vi "Find MAX Run.vi"(8 "error in (no error)":errorcluster, 10 "RUNSELECT (Most Recent, First, ALL)":string, 11 "Field Information":T1[](array[typedef])) -> (0 "error out":errorcluster, 3 "Field Information 2":T1[](array[typedef]))   [LabVIEW 2011]
uses:
  www/cgi-bin/_cgi-lib/TDM_INDEX Record.ctl
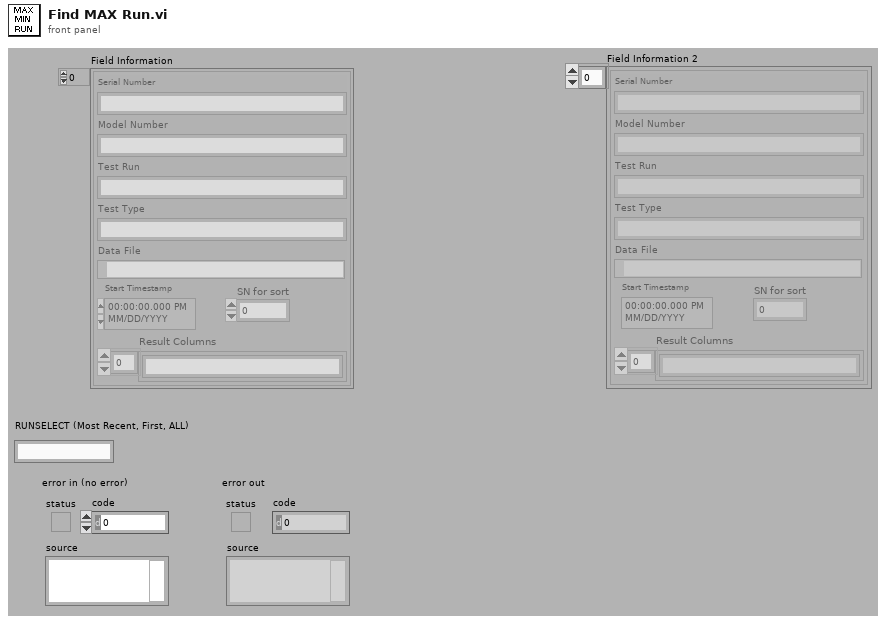
[diagram p1: front panel]
types:
  T1 = typedef "TDM_INDEX Record.ctl" = cluster{"Model Number":string, "SN for sort":i32, "Test Type":string, "Test Run":string, "Serial Number":string, "Start Timestamp":timestamp, "Data File":path, "Result Columns":string[]}
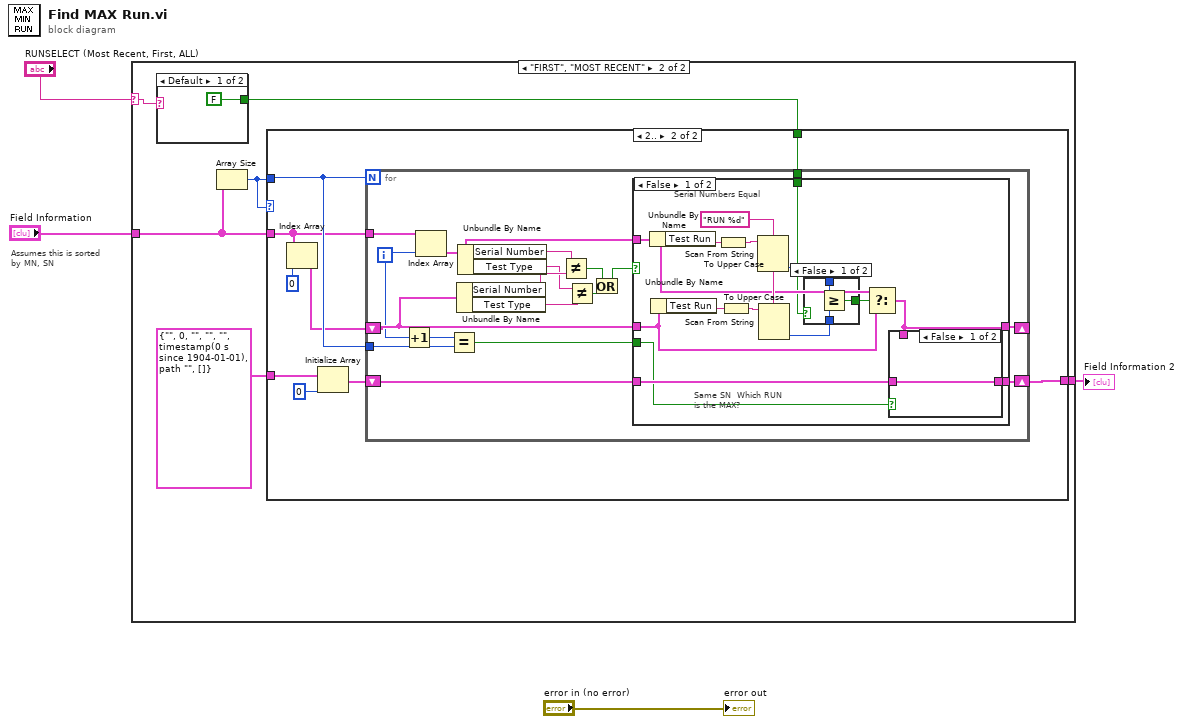
[diagram p0: block diagram]
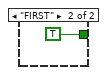
[diagram p3: hidden frame]
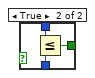
[diagram p5: hidden frame]
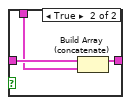
[diagram p6: hidden frame]
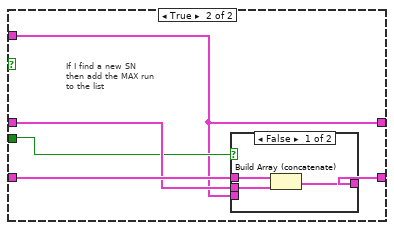
[diagram p7: hidden frame]
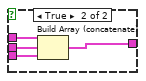
[diagram p8: hidden frame]
diagram:
  # "Assumes this is sorted \nby MN, SN"
  n1 = case shown="\"FIRST\", \"MOST RECENT\"" "RUNSELECT (Most Recent, First, ALL)" {
    selector: "RUNSELECT (Most Recent, First, ALL)" -> [_ w7]
    tunnel: [w5 w10] -> w3
    tunnel: "Field Information" -> [w5 w9]
    frame "ALL", Default {
    }
    frame "FIRST", "MOST RECENT" {
      n2 = case shown="Default" w7 {
        tunnel: [FALSE TRUE] -> w6
        frame Default {
        }
        frame "FIRST" {
        }
      }
      n3 = Array Size(array=w9) -> (size(s)=w8:i32)
      n4 = case shown="2.." w8 {
        tunnel: T1 {"Model Number"="", "SN for sort"=0, "Test Type"="", "Test Run"="", "Serial Number"="", "Start Timestamp"=timestamp(0 s since 1904-01-01), "Data File"=path "", "Result Columns"=[]} ("TDM_INDEX Record") -> [_ w23]
        tunnel: [w14 w20] -> w10
        tunnel: w9 -> [w14 w18]
        tunnel: w8 -> [_ w19]
        tunnel: w6 -> [_ w15]
        frame Default {
          # "If there are 0 or 1 elements no sorting is needed."
        }
        frame 2.. {
          n5 = Index Array(array=w18, index=0) -> (element=w16:T1)
          n6 = Initialize Array(w23, 0) -> (w21:T1[])
          n7 = for {
            N: w19 -> [_]
            shift-right: [w40] -> w20
            shift-left: w21 -> [w41]
            tunnel: w18 -> [w37]
            shift-right: [w38] -> _
            shift-left: w16 -> [w34]
            tunnel: w19 -> [w31]
            tunnel: w15 -> [w24]
            i -> [w32]
            n8 = Increment(x=w32) -> (x+1=w30:i32)
            n9 = Index Array(array=w37, index=w32) -> (element=w36:T1)
            n10 = Equal?(x=w30, y=w31) -> (x = y?=w35:bool)
            n11 = Unbundle By Name(w34) -> ("Serial Number"=w33:string, "Test Type"=w26:string)
            n12 = Unbundle By Name(w36) -> ("Serial Number"=w39:string, "Test Type"=w27:string)
            n13 = Not Equal?(x=w39, y=w33) -> (x != y?=w29:bool)
            n14 = Not Equal?(x=w27, y=w26) -> (x != y?=w25:bool)
            n15 = Or(x=w29, y=w25) -> (x .or. y?=w28:bool)
            n16 = case shown="False" w28 {
              tunnel: w41 -> [w50 w71]
              tunnel: [w51 w70] -> w40
              tunnel: w34 -> [w46 w69]
              tunnel: [w45 w67] -> w38
              tunnel: w36 -> [w47 w67]
              tunnel: w35 -> [w49 w68]
              tunnel: w24 -> [w42 _]
              frame False {
                w54 = "RUN %d" ("format string")
                # "Serial Numbers Equal"
                # "Same SN  Which RUN\nis the MAX?"
                n17 = Unbundle By Name(w47) -> ("Test Run"=w55:string)
                n18 = Unbundle By Name(w46) -> ("Test Run"=w56:string)
                n19 = To Upper Case(1:w55) -> (0:w44:string)
                n20 = To Upper Case(1:w56) -> (0:w43:string)
                n21 = Scan From String(format string=w54, input string=w44) -> (output 1=w53:i32)  [unwired: 2 in, 4 out]
                n22 = Scan From String(format string=w54, input string=w43) -> (output 1=w52:i32)  [unwired: 2 in, 4 out]
                n23 = case shown="False" w42 {
                  tunnel: w53 -> [w59 w62]
                  tunnel: w52 -> [w58 w61]
                  tunnel: [w57 w60] -> w48
                  frame False {
                    n24 = Greater Or Equal?(x=w59, y=w58) -> (x >= y?=w57:bool)
                  }
                  frame True {
                    n25 = Less Or Equal?(x=w62, y=w61) -> (x <= y?=w60:bool)
                  }
                }
                n26 = Select(t=w47, s=w48, f=w46) -> (s? t:f=w45:T1)
                n27 = case shown="False" w49 {
                  tunnel: [w63 w66] -> w51
                  tunnel: w50 -> [w63 w65]
                  tunnel: w45 -> [_ w64]
                  frame False {
                  }
                  frame True {
                    n28 = Build Array (concatenate)(w65, w64) -> (w66:T1[])
                  }
                }
              }
              frame True {
                # "If I find a new SN\nthen add the MAX run\nto the list"
                n29 = case shown="False" w68 {
                  tunnel: w71 -> [w74 w78]
                  tunnel: [w72 w77] -> w70
                  tunnel: w69 -> [w73 w76]
                  tunnel: w67 -> [_ w75]
                  frame False {
                    n30 = Build Array (concatenate)(w74, w73) -> (w72:T1[])
                  }
                  frame True {
                    n31 = Build Array (concatenate)(w78, w76, w75) -> (w77:T1[])
                  }
                }
              }
            }
          }
        }
      }
    }
  }
  "Field Information 2" <- w3
  "error out" <- "error in (no error)"
